vi "SVMabcFXP_src.vi"(0 "A":fxp<+/-,32,4>, 1 "max":fxp<+/-,32,4>=0.999969482421875 caption="max voltage", 5 "B":fxp<+/-,32,4>, 7 "C":fxp<+/-,32,4>) -> (4 "Upercent":fxp<+/-,32,4> caption="u voltage", 6 "Vpercent":fxp<+/-,32,4> caption="v voltage", 8 "Wpercent":fxp<+/-,32,4> caption="w voltage", 15 "Sector":u8)   [LabVIEW 2015]
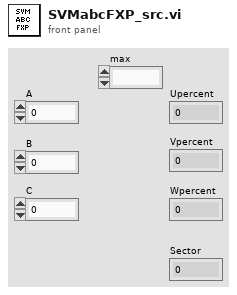
[diagram p1: front panel]
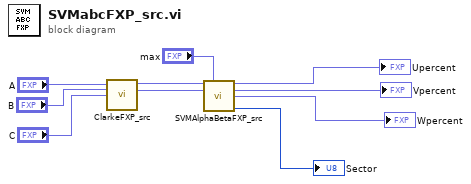
[diagram p0: block diagram]
diagram:
  n1 = call "ClarkeFXP_src.vi"("A"="A", "B"="B", "C"="C") -> ("alpha"=w10:fxp<+/-,32,4>, "beta"=w9:fxp<+/-,32,4>)  [unwired: 11 in]
  n2 = call "SVMAlphaBetaFXP_src.vi"("alpha"=w10, "max"="max", "beta"=w9) -> ("Upercent"=→"Upercent":fxp<+/-,32,4>, "Vpercent"=→"Vpercent":fxp<+/-,32,4>, "Wpercent"=→"Wpercent":fxp<+/-,32,4>, "Sector"=→"Sector":u8)  [unwired: 9 in]
